vi "tdms_read.vi"() -> ()   [LabVIEW 2021]
doc: "This example demonstrates how to benchmark the streaming performance when you use the TDMS Advanced Asynchronous I/O functions to read data from a .tdms file. This VI measures the time it takes to continuously read data from a file and calculates the average data throughput in bytes/second."
uses:
  specrogram_and_param.ctl
panel:
  out "time on secnario":dbl(slide) scale=0.0..36.7618529882353
  out "time in file":dbl
  out "# elements in queue":i32
  in  "Map selector":T1(ring)=enum."inverse grey"
  in  "center frequncy":dbl format="%#_6p"
  out "calculating":bool
  in  "reading time frame (sec)":dbl=1.0
  out "sampels per plot":ext format="%.2f"
  out "spectrogram":sgl[][](graph)
  out "fft size":ext
  in  "fft size in power of  2":i32=12
  in  "fs":dbl=20000000.0 format="%#_6p"
  in  "Next Button":bool
  in  "file path":path=path "C:/Users/NI/Documents/LabVIEW Data/streaming_test.tdms"
  # "TDMS file tester"
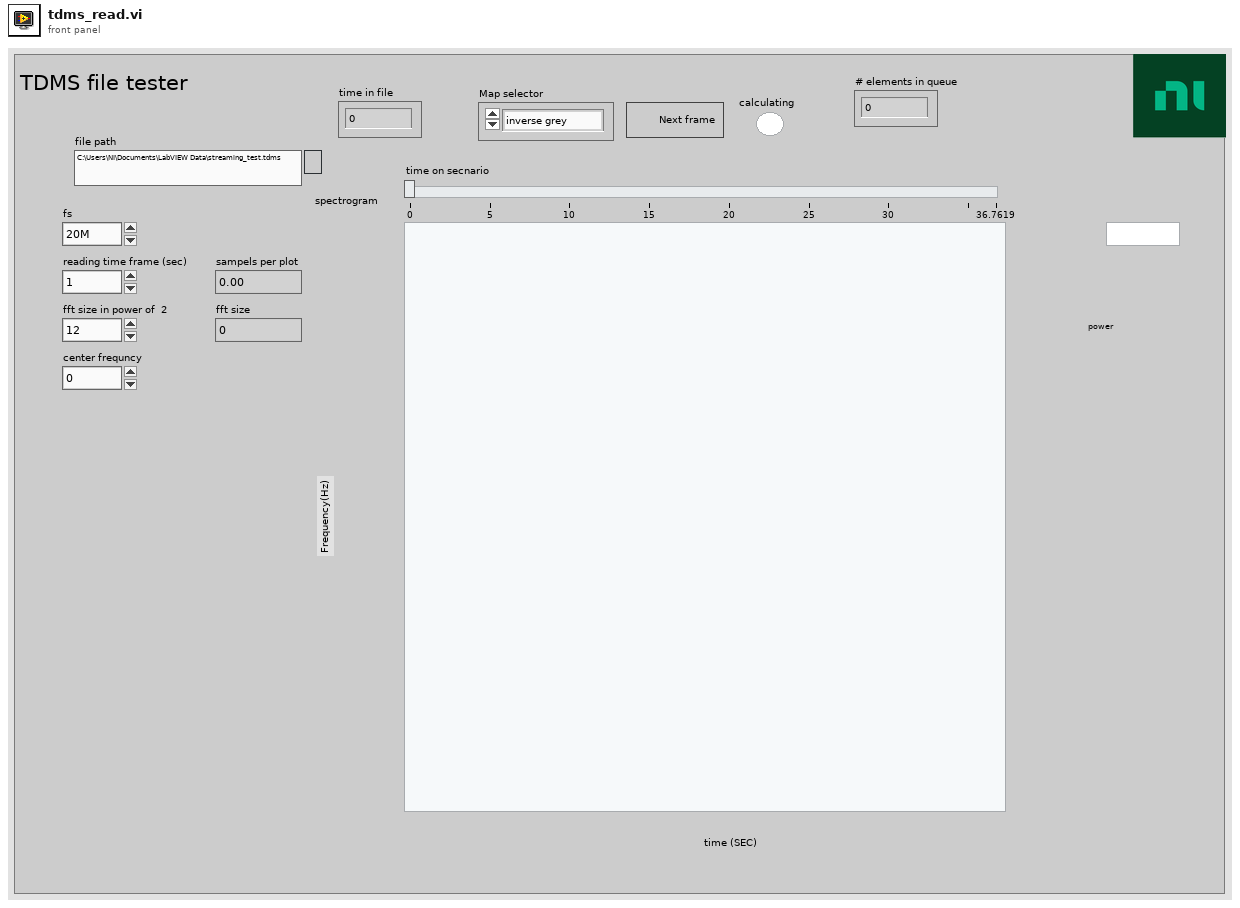
[diagram p1: front panel]
types:
  T1 = enum16{"fire", "rainbow", "grey", "inverse grey", "ice", "original"}
  T2 = typedef "specrogram_and_param.ctl" = cluster{"Array out":sgl[][], "start_ time":dbl, "min_amp":dbl, "amp_scale":dbl, "end of file":bool}
  T3 = enum16{"open", "open or create", "create or replace", "create", "open (read-only)"}
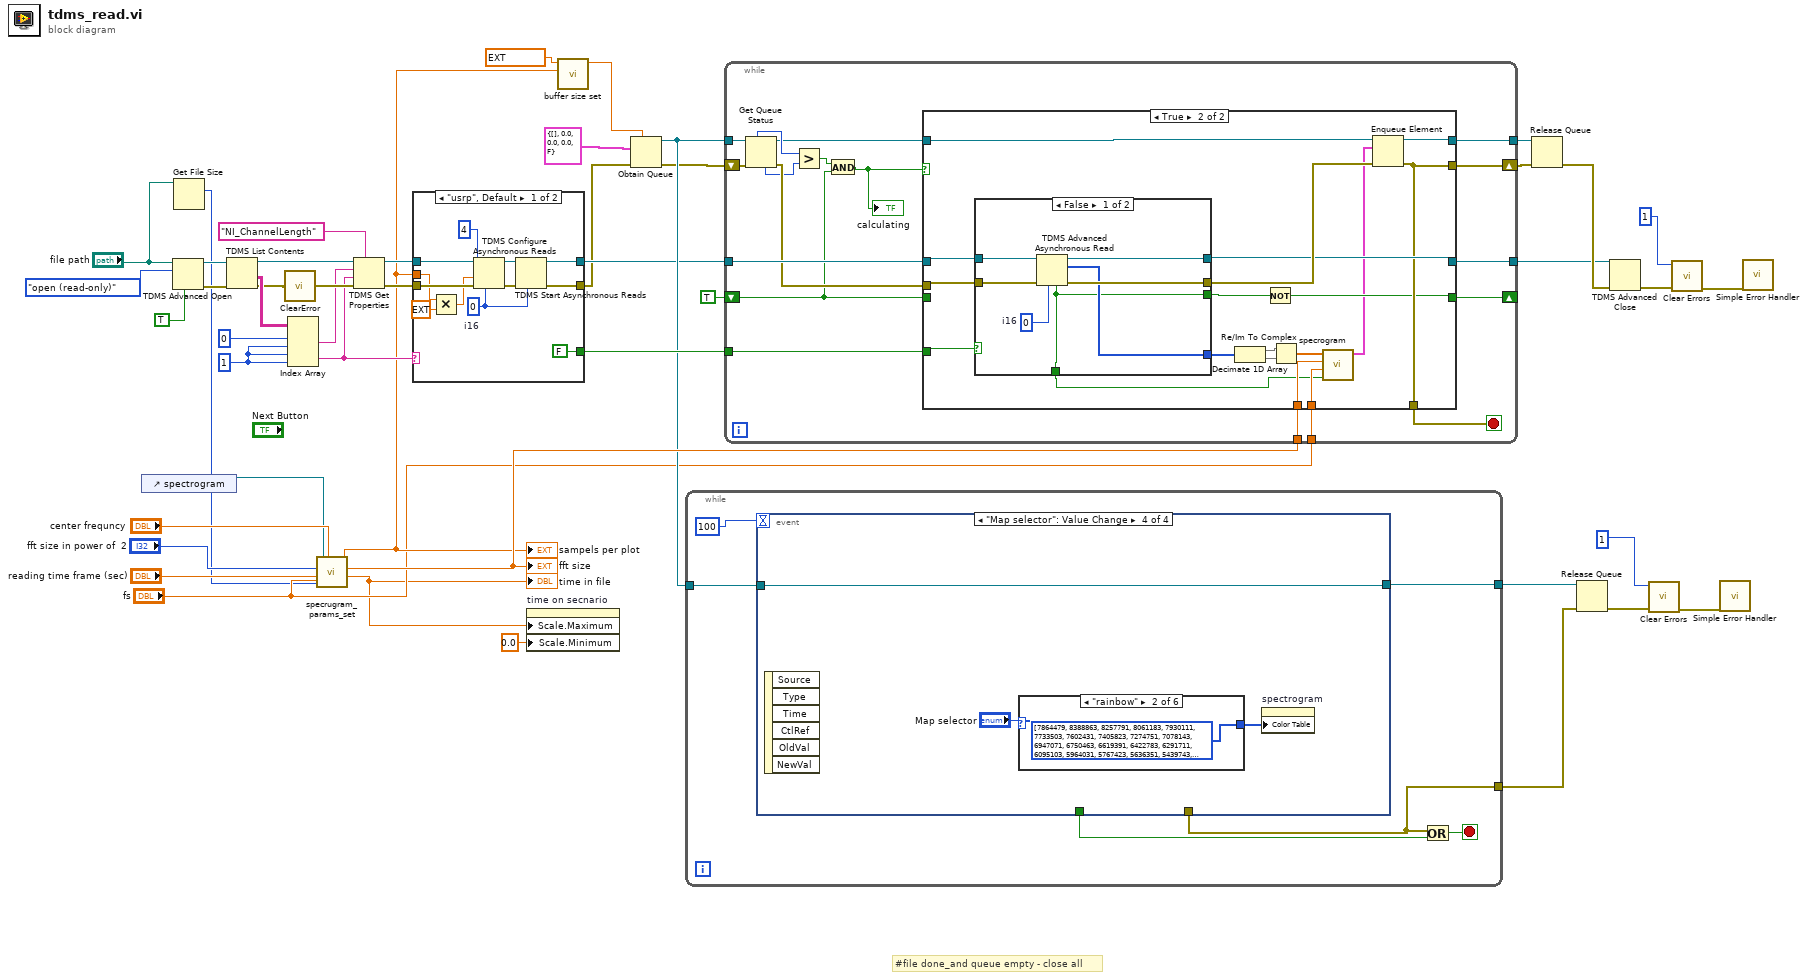
[diagram p0: block diagram]
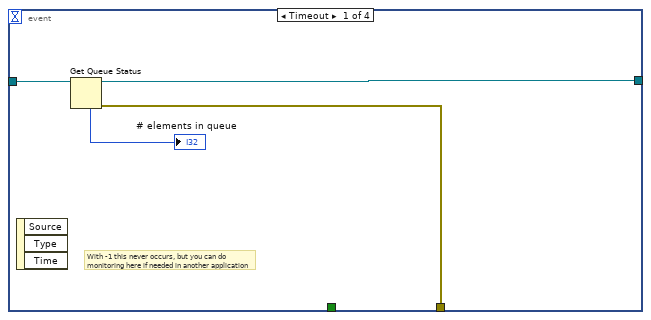
[diagram p2: hidden frame]
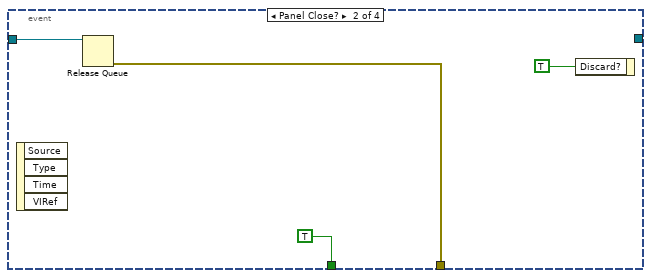
[diagram p3: hidden frame]
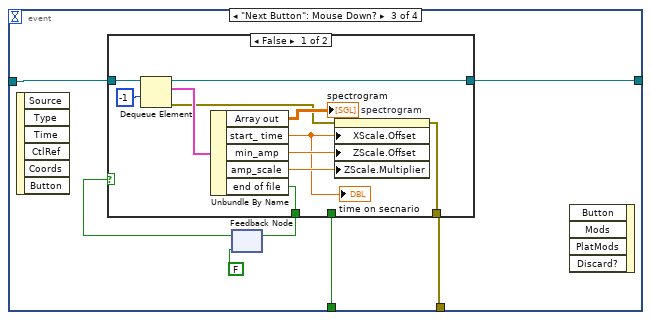
[diagram p4: hidden frame]
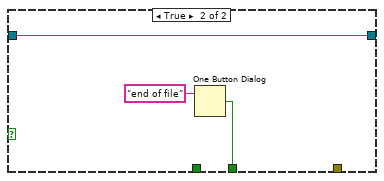
[diagram p5: hidden frame]
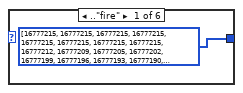
[diagram p6: hidden frame]
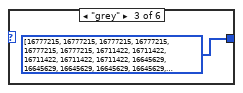
[diagram p7: hidden frame]
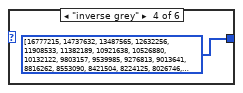
[diagram p8: hidden frame]
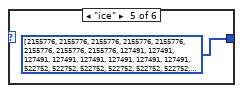
[diagram p9: hidden frame]
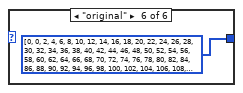
[diagram p10: hidden frame]
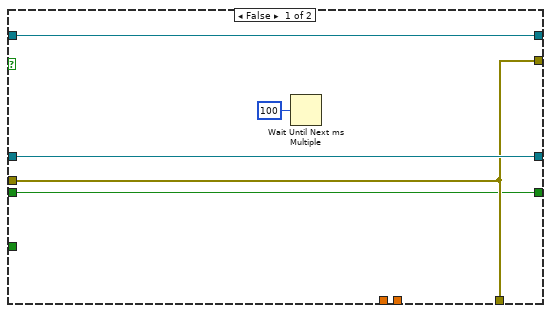
[diagram p11: hidden frame]
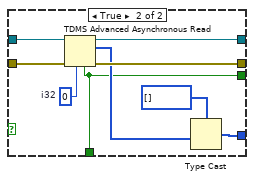
[diagram p12: hidden frame]
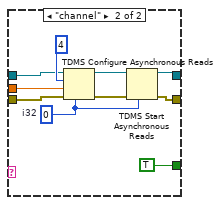
[diagram p13: hidden frame]
diagram:
  w44 = 1 ("disabled index (col)")
  # "#file done_and queue empty - close all"
  n1 = control-ref of="spectrogram"() -> (w19:refnum<vi>)
  n2 = TDMS Advanced Open(6:TRUE ("disable buffering? (T)"), 10:T3."open (read-only)" ("Operation"), 11:"file path") -> (0:w39:errorcluster, 3:w38:refnum<k34>)  [unwired: 2 in, 1 out]
  n3 = Get File Size(file="file path") -> (size (in bytes)=w4:i64)  [unwired: 1 in, 2 out]
  n4 = TDMS List Contents(4:w39, 7:w38) -> (0:w37:errorcluster, 1:w46:string[][], 3:w42:refnum<k34>)  [unwired: 1 in, 1 out]
  n5 = call <vilib>:"ClearError.vi"("error in (no error)"=w37) -> ("error out"=w43:errorcluster)
  n6 = Index Array(array=w46, index (row) #1=0 ("index (row)"), index (col) #1=w44, index (row) #2=w44, index (col) #2=w44) -> (element #1=w41:string, element #2=w34:string)
  n7 = call "specrugram_params_set.vi"("fs"="fs", "center frequncy"="center frequncy", "file size"=w4, "reading time frame (sec)"="reading time frame (sec)", "fft size in power of  in"="fft size in power of  2", 11:w19) -> ("time in file"=w3:dbl, "fft size"=w28:ext, "sampels per plot"=w6:ext)  [unwired: 1 in, 2 out]
  "sampels per plot" <- w6
  "fft size" <- w28
  "time in file" <- w3
  n8 = TDMS Get Properties(7:"NI_ChannelLength" ("property name"), 8:w43, 9:w34, 10:w41, 11:w42) -> (0:w33:errorcluster, 3:w32:refnum<k34>)  [unwired: 1 in, 4 out]
  n9 = case shown="\"usrp\", Default" w34 {
    tunnel: w33 -> [w56 w64]
    tunnel: w6 -> [w50 w61]
    tunnel: w32 -> [w53 w65]
    tunnel: [w54 w62] -> w25
    tunnel: [w52 w63] -> w24
    tunnel: [FALSE TRUE] -> w29
    frame "usrp", Default {
      w59 = i16 0  # i16
      n10 = Multiply(x=w50, y=ext 2.0) -> (x*y=w49:ext)
      n11 = TDMS Configure Asynchronous Reads(6:w59, 8:w56, 9:w49, 10:u32 4 ("number of buffers (4)"), 11:w53) -> (0:w57:errorcluster, 3:w58:refnum<k34>)  [unwired: 1 in]
      n12 = TDMS Start Asynchronous Reads(6:w59, 8:w57, 11:w58) -> (0:w52:errorcluster, 3:w54:refnum<k34>)  [unwired: 1 in]
    }
    frame "channel" {
      w69 = 0  # i32
      n13 = TDMS Configure Asynchronous Reads(6:w69, 8:w64, 9:w61, 10:u32 4 ("number of buffers (4)"), 11:w65) -> (0:w67:errorcluster, 3:w68:refnum<k34>)  [unwired: 1 in]
      n14 = TDMS Start Asynchronous Reads(6:w69, 8:w67, 11:w68) -> (0:w63:errorcluster, 3:w62:refnum<k34>)  [unwired: 1 in]
    }
  }
  n15 = property on="time on secnario" class="Slide (strict)"("Scale.Maximum"=w3, "Scale.Minimum"=0.0 ("Scale.Range:Minimum")) -> ()  [unwired: 2 in, 2 out]
  n16 = call "buffer size set.vi"("bytes per plot"=w6, "max number of sampels on the memory"=ext 100000000.0 ("y")) -> ("buffer size"=w15:ext)  [unwired: 9 in]
  n17 = Obtain Queue(max queue size (-1, unlimited)=w15, element data type=T2 {"Array out"=[], "start_ time"=0.0, "min_amp"=0.0, "amp_scale"=0.0, "end of file"=FALSE} ("Cluster"), error in (no error)=w24) -> (queue out=w26:refnum<queue>, error out=w23:errorcluster)  [unwired: 2 in, 1 out]
  n18 = while {
    tunnel: w26 -> [w74]
    tunnel: [w71] -> w12
    tunnel: [w73] -> w11
    stop <- w72 stop-if-true
    n19 = event shown="[3] \"Map selector\": Value Change" {
      selector: _ -> [_ _ _ _]
      dyn-events: _ -> [_ _ _ _]
      timeout: 100 ("Numeric") -> [_ _ _ _]
      tunnel: w74 -> [w79 w82 w85 w105]
      tunnel: [w77 w81 w90 _] -> w71
      tunnel: [w76 _ w84 w105] -> w73
      tunnel: [_ TRUE w86 _] -> w70
      event Timeout {
        # "With -1 this never occurs, but you can do monitoring here if needed in another application"
        n20 = event-data() -> ()  [unwired: 1 in, 3 out]
        n21 = Get Queue Status(queue=w79) -> (queue out=w76:refnum<queue>, error out=w77:errorcluster, # elements in queue=→"# elements in queue":i32)  [unwired: 2 in, 5 out]
      }
      event Panel Close? {
        n22 = event-data() -> ()  [unwired: 1 in, 4 out]
        n23 = Release Queue(queue=w82) -> (error out=w81:errorcluster)  [unwired: 2 in, 2 out]
        n24 = event-data("Discard?"=TRUE) -> ()  [unwired: 1 in, 1 out]
      }
      event "Next Button": Mouse Down? {
        n25 = event-data() -> ()  [unwired: 1 in, 6 out]
        n26 = feedback #1(FALSE ("end of file")) -> (w88:bool)
        n27 = case shown="False" w88 {
          tunnel: [w98 _] -> w90
          tunnel: [w96 _] -> w89
          tunnel: [_ w103] -> w86
          tunnel: w85 -> [w95 w102]
          tunnel: [w93 w102] -> w84
          frame False {
            n28 = Dequeue Element(queue=w95, timeout in ms (-1)=-1) -> (queue out=w93:refnum<queue>, element=w92:T2, error out=w91:errorcluster)  [unwired: 1 in, 1 out]
            n29 = Unbundle By Name(w92) -> ("Array out"=→"spectrogram":sgl[][], "start_ time"=w97:dbl, "min_amp"=w101:dbl, "amp_scale"=w100:dbl, "end of file"=w96:bool)
            "time on secnario" <- w97
            n30 = property on="spectrogram" class="IntGraph (strict)"(error in=w91, "XScale.Offset"=w97, "ZScale.Offset"=w101, "ZScale.Multiplier"=w100) -> (error out=w98:errorcluster)  [unwired: 1 in, 1 out]
          }
          frame True {
            n31 = One Button Dialog(message="end of file") -> (true=w103:bool)  [unwired: 1 in]
          }
        }
        n32 = feedback-in #1(w89) -> ()
        n33 = event-data() -> ()  [unwired: 5 in, 1 out]
      }
      event "Map selector": Value Change {
        n34 = event-data() -> ()  [unwired: 1 in, 6 out]
        n35 = case shown="\"rainbow\"" "Map selector" {
          tunnel: [u32[] [16777215, 16777215, 16777215, 16777215, 16777215, 16777215, 16777215, 16777215, 16777212, 16777209, 16777205, 16777202, 16777199, 16777196, 16777193, 16777190, 16777186, 16777183, 16777180, 16777177, 16777174, 16777170, 16777167, 16777164, 16777161, 16777158, 16777154, 16777151, 16777148, 16777145, 16777142, 16777139, 16777135, 16777132, 16777129, 16777126, 16777123, 16777119, 16777116, 16777113, 16777110, 16777107, 16777103, 16777100, 16777097, 16777094, 16777091, 16777088, 16777084, 16777081, 16777078, 16777075, 16777072, 16777068, 16777065, 16777062, 16777059, 16777056, 16777052, 16777049, 16777046, 16777043, 16777040, 16777037, 16777033, 16777030, 16777027, 16777024, 16777021, 16777017, 16777014, 16777011, 16777008, 16777005, 16777001, 16776998, 16776995, 16776992, 16776989, 16776986, 16776982, 16776979, 16776976, 16776973, 16776970, 16776966, 16776963, 16776960, 16776192, 16775424, 16774400, 16773632, 16772864, 16772096, 16771328, 16770560, 16769536, 16768768, 16768000, 16767232, 16766464, 16765440, 16764672, 16763904, 16763136, 16762368, 16761344, 16760576, 16759808, 16759040, 16758272, 16757504, 16756480, 16755712, 16754944, 16754176, 16753408, 16752384, 16751616, 16750848, 16750080, 16749312, 16748288, 16747520, 16746752, 16745984, 16745216, 16744448, 16743424, 16742656, 16741888, 16741120, 16740352, 16739328, 16738560, 16737792, 16737024, 16736256, 16735232, 16734464, 16733696, 16732928, 16732160, 16731392, 16730368, 16729600, 16728832, 16728064, 16727296, 16726272, 16725504, 16724736, 16723968, 16723200, 16722176, 16721408, 16720640, 16719872, 16719104, 16718336, 16717312, 16716544, 16715776, 16715008, 16714240, 16713216, 16712448, 16711680, 16515072, 16318464, 16056320, 15859712, 15663104, 15466496, 15269888, 15073280, 14811136, 14614528, 14417920, 14221312, 14024704, 13762560, 13565952, 13369344, 13172736, 12976128, 12713984, 12517376, 12320768, 12124160, 11927552, 11730944, 11468800, 11272192, 11075584, 10878976, 10682368, 10420224, 10223616, 10027008, 9830400, 9633792, 9371648, 9175040, 8978432, 8781824, 8585216, 8388608, 8126464, 7929856, 7733248, 7536640, 7340032, 7077888, 6881280, 6684672, 6488064, 6291456, 6029312, 5832704, 5636096, 5439488, 5242880, 5046272, 4784128, 4587520, 4390912, 4194304, 3997696, 3735552, 3538944, 3342336, 3145728, 2949120, 2686976, 2490368, 2293760, 2097152, 1900544, 1703936, 1441792, 1245184, 1048576, 851968, 655360, 393216, 196608, 65793, 65793, 65793, 65793, 65793, 65793, 65793, 65793, 0] ("256 fire") u32[] [7864479, 8388863, 8257791, 8061183, 7930111, 7733503, 7602431, 7405823, 7274751, 7078143, 6947071, 6750463, 6619391, 6422783, 6291711, 6095103, 5964031, 5767423, 5636351, 5439743, 5308671, 5112063, 4980991, 4784383, 4653311, 4456703, 4325631, 4129023, 3932415, 3801343, 3604735, 3473663, 3277055, 3145983, 2949375, 2818303, 2621695, 2490623, 2294015, 2162943, 1966335, 1835263, 1638655, 1507583, 1310975, 1179903, 983295, 852223, 655615, 524543, 327935, 196863, 511, 1791, 3071, 4351, 5631, 6911, 8191, 9471, 10751, 12031, 13311, 14591, 15871, 17151, 18431, 19711, 20991, 22271, 23551, 24831, 26111, 27391, 28671, 29951, 31231, 32511, 33791, 35071, 36351, 37631, 38911, 40191, 41471, 42751, 44031, 45311, 46591, 47871, 49151, 50431, 51711, 52991, 54271, 55551, 56831, 58111, 59391, 60671, 61951, 63231, 64511, 65532, 65527, 65522, 65517, 65512, 65507, 65502, 65497, 65492, 65487, 65482, 65477, 65472, 65467, 65462, 65457, 65452, 65447, 65442, 65437, 65432, 65427, 65422, 65417, 65412, 65407, 65402, 65397, 65392, 65387, 65382, 65377, 65372, 65367, 65362, 65357, 65352, 65347, 65342, 65337, 65332, 65327, 65322, 65317, 65312, 65307, 65302, 65297, 65292, 65287, 65282, 261888, 589568, 917248, 1244928, 1572608, 1900288, 2227968, 2555648, 2883328, 3211008, 3538688, 3866368, 4194048, 4521728, 4849408, 5177088, 5504768, 5832448, 6160128, 6487808, 6815488, 7143168, 7470848, 7798528, 8126208, 8453888, 8781568, 9109248, 9436928, 9764608, 10092288, 10419968, 10747648, 11075328, 11403008, 11730688, 12058368, 12386048, 12713728, 13041408, 13369088, 13696768, 14024448, 14352128, 14679808, 15007488, 15335168, 15662848, 15990528, 16318208, 16645888, 16775936, 16774656, 16773376, 16772096, 16770816, 16769536, 16768256, 16766976, 16765696, 16764416, 16763136, 16761856, 16760576, 16759296, 16758016, 16756736, 16755456, 16754176, 16752896, 16751616, 16750336, 16749056, 16747776, 16746496, 16745216, 16743936, 16742656, 16741376, 16740096, 16738816, 16737536, 16736256, 16734976, 16733696, 16732416, 16731136, 16729856, 16728576, 16727296, 16726016, 16724736, 16723456, 16722176, 16720896, 16719616, 16718336, 16717056, 16715776, 16714496, 16713216, 16711680] ("rainbow") u32[] [16777215, 16777215, 16777215, 16777215, 16777215, 16777215, 16711422, 16711422, 16711422, 16711422, 16711422, 16645629, 16645629, 16645629, 16645629, 16645629, 16645629, 16579836, 16579836, 16579836, 16579836, 16579836, 16514043, 16514043, 16514043, 16514043, 16514043, 16448250, 16448250, 16448250, 16448250, 16448250, 16316664, 16382457, 16382457, 16382457, 16382457, 16316664, 16316664, 16316664, 16316664, 16250871, 16250871, 16250871, 16250871, 16250871, 16185078, 16185078, 16185078, 16185078, 16119285, 16119285, 16119285, 16119285, 16119285, 16053492, 16053492, 16053492, 16053492, 15987699, 15987699, 15987699, 15987699, 15921906, 15987699, 15921906, 15921906, 15856113, 15856113, 15856113, 15856113, 15856113, 15790320, 15790320, 15790320, 15724527, 15724527, 15724527, 15724527, 15658734, 15658734, 15658734, 15658734, 15592941, 15592941, 15592941, 15592941, 15527148, 15527148, 15527148, 15461355, 15461355, 15461355, 15461355, 15395562, 15395562, 15395562, 15395562, 15329769, 15329769, 15329769, 15263976, 15263976, 15263976, 15198183, 15198183, 15198183, 15198183, 15132390, 15132390, 15132390, 15066597, 15066597, 15066597, 15000804, 15000804, 15000804, 14935011, 14935011, 14935011, 14869218, 14869218, 14869218, 14803425, 14803425, 14803425, 14737632, 14737632, 14671839, 14671839, 14671839, 14606046, 14606046, 14606046, 14540253, 14540253, 14540253, 14474460, 14474460, 14408667, 14408667, 14408667, 14342874, 14342874, 14277081, 14277081, 14277081, 14211288, 14211288, 14145495, 14145495, 14079702, 14079702, 14013909, 14013909, 14013909, 13948116, 13948116, 13882323, 13882323, 13816530, 13816530, 13750737, 13750737, 13684944, 13684944, 13619151, 13619151, 13553358, 13553358, 13487565, 13487565, 13421772, 13421772, 13355979, 13290186, 13290186, 13224393, 13224393, 13158600, 13092807, 13092807, 13027014, 13027014, 12961221, 12895428, 12895428, 12829635, 12763842, 12763842, 12698049, 12632256, 12566463, 12566463, 12500670, 12434877, 12434877, 12369084, 12303291, 12237498, 12171705, 12171705, 12105912, 12040119, 11974326, 11908533, 11842740, 11776947, 11711154, 11645361, 11579568, 11513775, 11447982, 11382189, 11316396, 11250603, 11184810, 11119017, 10987431, 10921638, 10855845, 10790052, 10658466, 10592673, 10461087, 10395294, 10329501, 10197915, 10066329, 10000536, 9868950, 9737364, 9605778, 9474192, 9342606, 9211020, 9079434, 8882055, 8750469, 8553090, 8421504, 8224125, 7960953, 7763574, 7500402, 7237230, 6974058, 6645093, 6316128, 5855577, 5395026, 4868682, 4210752, 3289650, 2105376, 0] ("256 log up") u32[] [16777215, 14737632, 13487565, 12632256, 11908533, 11382189, 10921638, 10526880, 10132122, 9803157, 9539985, 9276813, 9013641, 8816262, 8553090, 8421504, 8224125, 8026746, 7895160, 7697781, 7566195, 7434609, 7303023, 7171437, 7039851, 6908265, 6776679, 6710886, 6579300, 6447714, 6381921, 6316128, 6184542, 6118749, 5987163, 5921370, 5855577, 5789784, 5658198, 5592405, 5526612, 5460819, 5395026, 5329233, 5263440, 5197647, 5131854, 5066061, 5000268, 4934475, 4868682, 4802889, 4737096, 4671303, 4605510, 4605510, 4539717, 4473924, 4408131, 4342338, 4342338, 4276545, 4210752, 4210752, 4144959, 4079166, 4013373, 4013373, 3947580, 3881787, 3881787, 3815994, 3750201, 3750201, 3684408, 3684408, 3618615, 3552822, 3552822, 3487029, 3487029, 3421236, 3421236, 3355443, 3289650, 3289650, 3223857, 3223857, 3158064, 3158064, 3092271, 3092271, 3026478, 3026478, 2960685, 2960685, 2894892, 2894892, 2829099, 2829099, 2763306, 2763306, 2763306, 2697513, 2697513, 2631720, 2631720, 2565927, 2565927, 2500134, 2500134, 2500134, 2434341, 2434341, 2368548, 2368548, 2368548, 2302755, 2302755, 2236962, 2236962, 2236962, 2171169, 2171169, 2171169, 2105376, 2105376, 2105376, 2039583, 2039583, 1973790, 1973790, 1973790, 1907997, 1907997, 1907997, 1842204, 1842204, 1842204, 1776411, 1776411, 1776411, 1710618, 1710618, 1710618, 1644825, 1644825, 1644825, 1579032, 1579032, 1579032, 1579032, 1513239, 1513239, 1513239, 1447446, 1447446, 1447446, 1381653, 1381653, 1381653, 1381653, 1315860, 1315860, 1315860, 1315860, 1250067, 1250067, 1250067, 1184274, 1184274, 1184274, 1184274, 1118481, 1118481, 1118481, 1118481, 1052688, 1052688, 1052688, 1052688, 986895, 986895, 986895, 921102, 921102, 921102, 921102, 921102, 855309, 855309, 855309, 855309, 789516, 789516, 789516, 789516, 723723, 723723, 723723, 723723, 657930, 657930, 657930, 657930, 657930, 592137, 592137, 592137, 592137, 526344, 526344, 526344, 526344, 526344, 460551, 460551, 460551, 460551, 460551, 394758, 394758, 394758, 394758, 328965, 328965, 328965, 328965, 328965, 263172, 263172, 263172, 263172, 263172, 197379, 197379, 197379, 197379, 197379, 131586, 131586, 131586, 131586, 131586, 131586, 65793, 65793, 65793, 65793, 65793, 0, 0, 0, 0, 0, 0] ("256 log down") u32[] [2155776, 2155776, 2155776, 2155776, 2155776, 2155776, 2155776, 2155776, 127491, 127491, 127491, 127491, 127491, 127491, 127491, 127491, 522752, 522752, 522752, 522752, 522752, 522752, 522752, 522752, 64018, 64018, 64018, 64018, 64018, 64018, 64018, 64018, 63778, 63778, 63778, 63778, 63778, 63778, 63778, 63778, 63790, 63790, 63790, 63790, 63790, 63790, 63790, 63790, 63797, 63797, 63797, 63797, 63797, 63797, 63797, 63797, 63807, 63807, 63807, 63807, 63807, 63807, 63807, 63807, 64068, 64068, 64068, 64068, 64068, 64068, 64068, 64068, 63828, 63828, 63828, 63828, 63828, 63828, 63828, 63828, 63833, 63833, 63833, 63833, 63833, 63833, 63833, 63833, 63836, 63836, 63836, 63836, 63836, 63836, 63836, 63836, 63836, 63836, 63836, 63836, 63836, 63836, 63836, 63836, 61790, 61790, 61790, 61790, 61790, 61790, 61790, 61790, 58464, 58464, 58464, 58464, 58464, 58464, 58464, 58464, 55387, 55387, 55387, 55387, 55387, 55387, 55387, 55387, 51286, 51286, 51286, 51286, 51286, 51286, 51286, 51286, 47440, 47440, 47440, 47440, 47440, 47440, 47440, 47440, 40284, 40284, 40284, 40284, 40284, 40284, 40284, 40284, 34154, 34154, 34154, 34154, 34154, 34154, 34154, 34154, 28540, 28540, 28540, 28540, 28540, 28540, 28540, 28540, 20113, 20113, 20113, 20113, 20113, 20113, 20113, 20113, 12193, 12193, 12193, 12193, 12193, 12193, 12193, 12193, 12714, 12714, 12714, 12714, 12714, 12714, 12714, 12714, 7351, 7351, 7351, 7351, 7351, 7351, 7351, 7351, 4800, 4800, 4800, 4800, 4800, 4800, 4800, 4800, 195, 195, 195, 195, 195, 195, 195, 195, 189, 189, 189, 189, 189, 189, 189, 189, 183, 183, 183, 183, 183, 183, 183, 183, 175, 175, 175, 175, 175, 175, 175, 175, 164, 164, 164, 164, 164, 164, 164, 164, 155, 155, 155, 155, 155, 155, 155, 155] ("32 ice") u32[] [0, 0, 2, 4, 6, 8, 10, 12, 14, 16, 18, 20, 22, 24, 26, 28, 30, 32, 34, 36, 38, 40, 42, 44, 46, 48, 50, 52, 54, 56, 58, 60, 62, 64, 66, 68, 70, 72, 74, 76, 78, 80, 82, 84, 86, 88, 90, 92, 94, 96, 98, 100, 102, 104, 106, 108, 110, 112, 114, 116, 118, 120, 122, 124, 126, 128, 130, 132, 134, 136, 138, 140, 142, 144, 146, 148, 150, 152, 154, 156, 158, 160, 162, 164, 166, 168, 170, 172, 174, 176, 178, 180, 182, 184, 186, 188, 190, 192, 194, 196, 198, 200, 202, 204, 206, 208, 210, 212, 214, 216, 218, 220, 222, 224, 226, 228, 230, 232, 234, 236, 238, 240, 242, 244, 246, 248, 250, 252, 255, 131839, 263423, 395007, 526591, 658175, 789759, 921343, 1052927, 1184511, 1316095, 1447679, 1579263, 1710847, 1842431, 1974015, 2105599, 2237183, 2368767, 2500351, 2631935, 2763519, 2895103, 3026687, 3158271, 3289855, 3421439, 3553023, 3684607, 3816191, 3947775, 4079359, 4210943, 4342527, 4474111, 4605695, 4737279, 4868863, 5000447, 5132031, 5263615, 5395199, 5526783, 5658367, 5789951, 5921535, 6053119, 6184703, 6316287, 6447871, 6579455, 6711039, 6842623, 6974207, 7105791, 7237375, 7368959, 7500543, 7632127, 7763711, 7895295, 8026879, 8158463, 8290047, 8421631, 8553215, 8684799, 8816383, 8947967, 9079551, 9211135, 9342719, 9474303, 9605887, 9737471, 9869055, 10000639, 10132223, 10263807, 10395391, 10526975, 10658559, 10790143, 10921727, 11053311, 11184895, 11316479, 11448063, 11579647, 11711231, 11842815, 11974399, 12105983, 12237567, 12369151, 12500735, 12632319, 12763903, 12895487, 13027071, 13158655, 13290239, 13421823, 13553407, 13684991, 13816575, 13948159, 14079743, 14211327, 14342911, 14474495, 14606079, 14737663, 14869247, 15000831, 15132415, 15263999, 15395583, 15527167, 15658751, 15790335, 15921919, 16053503, 16185087, 16316671, 16448255, 16579839, 16777215] ("original")] -> w106
          frame .."fire" {
          }
          frame "rainbow" {
          }
          frame "grey" {
          }
          frame "inverse grey" {
          }
          frame "ice" {
          }
          frame "original" {
          }
        }
        n36 = property on="spectrogram" class="IntGraph (strict)"("Color Table"=w106) -> ()  [unwired: 2 in, 2 out]
      }
    }
    n37 = Or(x=w71, y=w70) -> (x .or. y?=w72:bool)
  }
  n38 = while {
    tunnel: w25 -> [w131]
    tunnel: w29 -> [w130]
    tunnel: w28 -> [w129]
    shift-right: [w120] -> w22
    shift-left: w23 -> [w123]
    tunnel: w26 -> [w128]
    tunnel: "fs" -> [w125]
    tunnel: [w124] -> w27
    tunnel: [w121] -> w20
    shift-right: [w119] -> _
    shift-left: TRUE -> [w116]
    stop <- w114 stop-if-true
    n39 = Get Queue Status(queue=w128, error in (no error)=w123) -> (queue out=w126:refnum<queue>, max queue size=w127:i32, error out=w122:errorcluster, # elements in queue=w115:i32)  [unwired: 1 in, 4 out]
    n40 = Greater?(x=w127, y=w115) -> (0:w118:bool)
    n41 = And(x=w118, y=w116) -> (x .and. y?=w117:bool)
    "calculating" <- w117
    n42 = case shown="True" w117 {
      tunnel: w131 -> [w134 w154]
      tunnel: w130 -> [_ w153]
      tunnel: w122 -> [w133 w152]
      tunnel: [w133 w141] -> w120
      tunnel: w129 -> [_ w151]
      tunnel: w126 -> [w135 w146]
      tunnel: w125 -> [_ w145]
      tunnel: [w135 w144] -> w124
      tunnel: [w134 w142] -> w121
      tunnel: [w133 w141] -> w114
      tunnel: [w132 w139] -> w119
      tunnel: w116 -> [w132 _]
      frame False {
        n43 = Wait Until Next ms Multiple(millisecond multiple=u32 100) -> ()  [unwired: 1 out]
      }
      frame True {
        n44 = case shown="False" w153 {
          tunnel: [w159 w170] -> w150
          tunnel: [w161 w168] -> w143
          tunnel: [w160 w167] -> w142
          tunnel: w154 -> [w157 w164]
          tunnel: w152 -> [w156 w163]
          tunnel: [w155 w162] -> w140
          tunnel: [w155 w162] -> w138
          frame False {
            w158 = i16 0  # i16
            n45 = TDMS Advanced Asynchronous Read(6:w158, 8:w156, 11:w157) -> (0:w161:errorcluster, 2:w159:i16[], 3:w160:refnum<k34>, 4:w155:bool)
          }
          frame True {
            w166 = 0  # i32
            n46 = TDMS Advanced Asynchronous Read(6:w166, 8:w163, 11:w164) -> (0:w168:errorcluster, 2:w165:i32[], 3:w167:refnum<k34>, 4:w162:bool)
            n47 = Type Cast(type=i16[] [], x=w165) -> (*(type *) &x=w170:i16[])
          }
        }
        n48 = Decimate 1D Array(w150) -> (w149:i16[], w148:i16[])
        n49 = Not(x=w140) -> (.not. x?=w139:bool)
        n50 = Re/Im To Complex(1:w148, 2:w149) -> (0:w147:cdb[])
        n51 = call "specrogram.vi"("end of file"=w138, "Fs"=w145, "fft size"=w151, "Array in"=w147) -> ("specrogram"=w137:T2)  [unwired: 7 in]
        n52 = Enqueue Element(queue=w146, element=w137, error in (no error)=w143) -> (queue out=w144:refnum<queue>, error out=w141:errorcluster)  [unwired: 1 in, 1 out]
      }
    }
  }
  n53 = Release Queue(queue=w27, error in (no error)=w22) -> (error out=w21:errorcluster)  [unwired: 1 in, 2 out]
  n54 = Release Queue(queue=w11, error in (no error)=w12) -> (error out=w9:errorcluster)  [unwired: 1 in, 2 out]
  n55 = TDMS Advanced Close(8:w21, 11:w20) -> (0:w18:errorcluster)  [unwired: 2 in, 1 out]
  n56 = call <vilib>:"Clear Errors.vi"("error in (no error)"=w9, "specific error code to clear (0: all)"=1) -> ("error out"=w10:errorcluster)  [unwired: 4 in, 1 out]
  n57 = call <vilib>:"Clear Errors.vi"("error in (no error)"=w18, "specific error code to clear (0: all)"=1) -> ("error out"=w17:errorcluster)  [unwired: 4 in, 1 out]
  n58 = call <vilib>:"Simple Error Handler.vi"("error in (no error)"=w10) -> ()  [unwired: 1 in, 8 out]
  n59 = call <vilib>:"Simple Error Handler.vi"("error in (no error)"=w17) -> ()  [unwired: 1 in, 8 out]
